vi "Write Data.vi"(7 "TX.Data":T1 caption="Transmission Data" format="%.0x", 8 "error in (no error)":errorcluster, 11 "Low Speed in":refnum<class "Low Speed.lvclass">) -> (0 "error out":errorcluster, 3 "Low Speed out":refnum<class "Low Speed.lvclass">)   [LabVIEW 2020, in "Low Speed.lvclass"]
uses:
  Low Speed.lvclass
  C:/Users/kaiser.asan/OneDrive - SolitonTechnologies/LabVIEW/29.SDLC - I2C Driver/I2C Module/I2C Controller Module/Class/Transmission Mode/Parent/TX Speed.lvclass
  TypeDef/Transmission Data.ctl
  Low Speed.lvclass/Low Speed.ctl
  Parent/TX Speed.lvclass
  I2C Controller Lib.lvlib
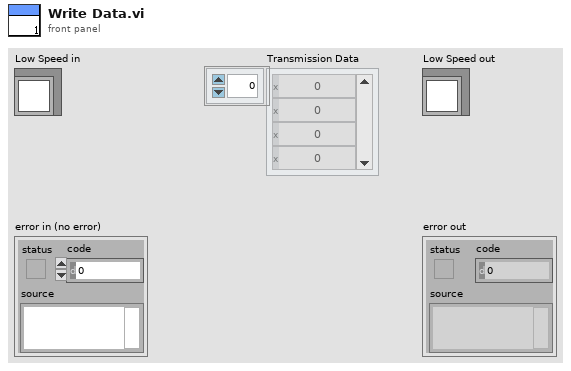
[diagram p1: front panel]
types:
  T1 = typedef "I2C Controller Lib.lvlib/Transmission Data.ctl" = u8[]
  T2 = typedef "I2C Controller Lib.lvlib/Timing Parameters Cluster.ctl" = cluster{"f_SCL(KHz)":u32, "t_HIGH (ns)":u32, "t_LOW (ns)":u32, "t_SU;STA (ns)":u32, "t_HD;STA (ns)":u32, "t_SU;DAT (ns)":u32, "t_HD;DAT (ns)":u32, "t_SU;STO (ns)":u32, "t_BUF (ns)":u32}
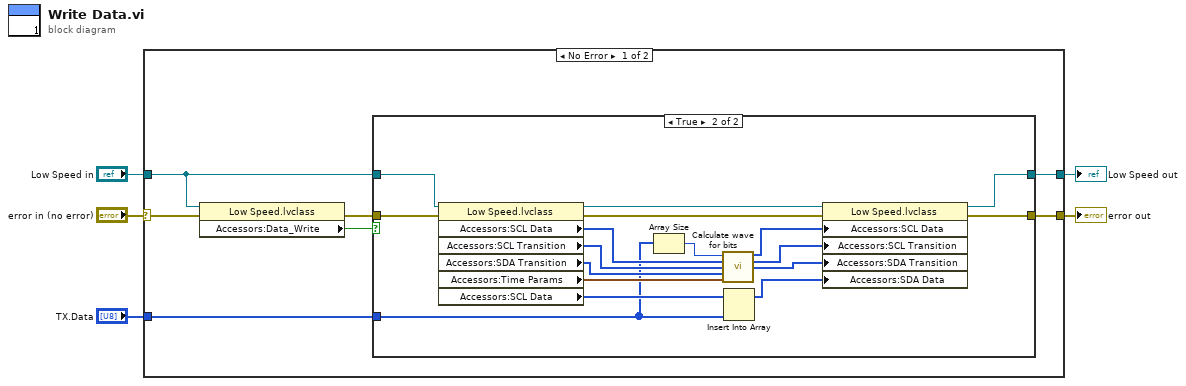
[diagram p0: block diagram]
diagram:
  n1 = case shown="No Error" "error in (no error)" {
    selector: "error in (no error)" -> [w12 w33]
    tunnel: [w11 w33] -> w5
    tunnel: [w9 w32] -> w3
    tunnel: "Low Speed in" -> [w8 w32]
    tunnel: "TX.Data" -> [w6 _]
    frame No Error {
      n2 = property class="Low Speed.lvclass"(reference=w8, error in=w12) -> (error out=w10:errorcluster, "Accessors:Data_Write"=w7:bool)  [unwired: 1 out]
      n3 = case shown="True" w7 {
        tunnel: [w13 w29] -> w11
        tunnel: w10 -> [w13 w31]
        tunnel: [w14 w27] -> w9
        tunnel: w8 -> [w14 w26]
        tunnel: w6 -> [_ w15]
        frame False {
        }
        frame True {
          n4 = property class="Low Speed.lvclass"(reference=w26, error in=w31) -> (reference out=w28:refnum<class "Low Speed.lvclass">, error out=w30:errorcluster, "Accessors:SCL Data"=w25:u8[], "Accessors:SCL Transition"=w24:u32[], "Accessors:SDA Transition"=w23:u32[], "Accessors:Time Params"=w22:T2, "Accessors:SCL Data"=w18:u8[])
          n5 = Array Size(array=w15) -> (size(s)=w16:i32)
          n6 = call "Calculate wave for bits.vi"("No. Of Bits"=w16, "SCL DATA IN"=w25, "SCL Transitions In"=w24, "SDA Transitions In"=w23, "Time Params"=w22) -> ("SCL DATA OUT"=w21:u8[], "SCL Transitions Out"=w20:u32[], "SDA Transitions Out"=w19:u32[])  [unwired: 8 in]
          n7 = Insert Into Array(array=w18, new element=w15) -> (w17:u8[])  [unwired: 1 in]
          n8 = property class="Low Speed.lvclass"(reference=w28, error in=w30, "Accessors:SCL Data"=w21, "Accessors:SCL Transition"=w20, "Accessors:SDA Transition"=w19, "Accessors:SDA Data"=w17) -> (reference out=w27:refnum<class "Low Speed.lvclass">, error out=w29:errorcluster)
        }
      }
    }
    frame Error {
    }
  }
  "error out" <- w5
  "Low Speed out" <- w3
